vi "UPPub.vi"(8 "error in (no error)":errorcluster, 11 "GuiderSetup in":refnum<class "GuiderSetup.lvclass">) -> (0 "error out":errorcluster, 2 "STATUS cluster":T1, 3 "GuiderSetup out":refnum<class "GuiderSetup.lvclass">)   [LabVIEW 2018, in "GuiderSetup.lvclass"]
uses:
  GuiderSetup.lvclass
  C:/Users/observer/Desktop/Sparc4GUI/Versao ZeroMQ/SPARC4_GUI -20240706_20240708/S4GUI/S4GUI.lvclass
  S4GUI/S4GUI.lvclass/S4GUI.ctl
  Server/Server.lvclass/Server.ctl
  GuiderSetup.lvclass/GuiderSetup.ctl
  Instrument/Instrument.lvclass
  C:/Users/observer/Desktop/Sparc4GUI/Versao ZeroMQ/SPARC4_GUI -20240706_20240708/Server/Server.lvclass
  PublisherGS/PublisherGS.lvclass
  AG/AG.lvclass
  Server/Server.lvclass
  S4GUI/S4GUI.lvclass
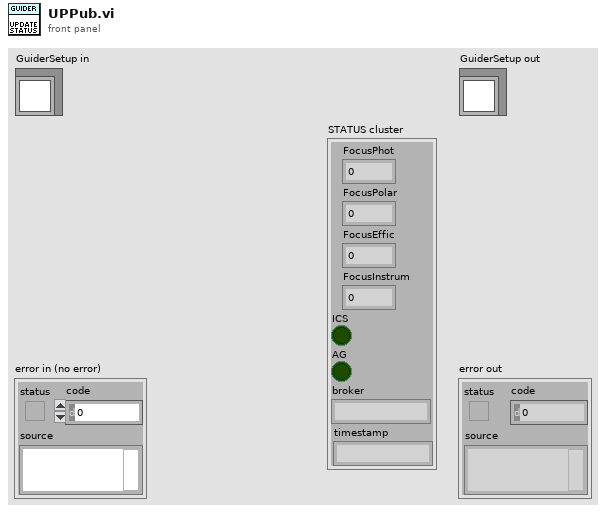
[diagram p1: front panel]
types:
  T1 = cluster{"FocusPhot":dbl, "FocusPolar":dbl, "FocusEffic":dbl, "FocusInstrum":dbl, "ICS":bool, "AG":bool, "broker":string, "timestamp":string}
  T2 = cluster{"Photometric":dbl, " Polarimetry":dbl, "Polarimetry \nEfficiency":dbl, "Instrumental polarization":dbl}
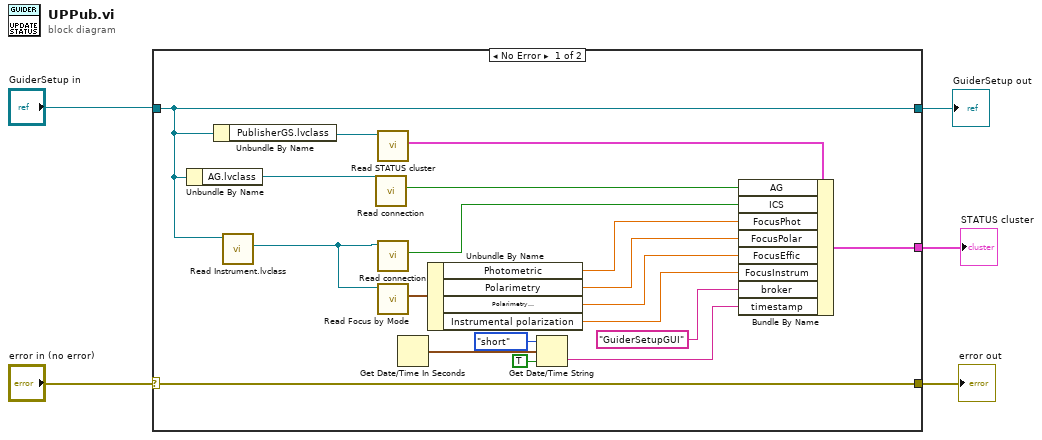
[diagram p0: block diagram]
diagram:
  n1 = case shown="No Error" "error in (no error)" {
    selector: "error in (no error)" -> [w10 w25]
    tunnel: [w19 w26] -> w2
    tunnel: "GuiderSetup in" -> [w19 w26]
    tunnel: [w24 _] -> w1
    tunnel: [w10 w25] -> w3
    frame No Error {
      n2 = Unbundle By Name(w19) -> ("AG.lvclass"=w21:refnum<class "AG.lvclass">)
      n3 = Unbundle By Name(w19) -> ("PublisherGS.lvclass"=w23:refnum<class "PublisherGS.lvclass">)
      n4 = call "Read Instrument.lvclass.vi"("S4ACS_GUI in"=w19) -> ("Instrument.lvclass"=w17:refnum<class "Instrument.lvclass">)  [unwired: 8 in, 2 out]
      n5 = call-dynamic "Read connection.vi"("Client in"=w21) -> ("connection"=w20:bool)  [unwired: 8 in, 2 out]
      n6 = call-dynamic "Read STATUS cluster.vi"("PublisherGS in"=w23) -> ("STATUS cluster"=w22:T1)  [unwired: 8 in, 2 out]
      n7 = call "Read connection.vi"("Server in"=w17) -> ("connection"=w18:bool)  [unwired: 8 in, 2 out]
      n8 = call-dynamic "Read Focus by Mode.vi"("Instrument in"=w17) -> ("Focus by Mode"=w16:T2)  [unwired: 8 in, 2 out]
      n9 = Get Date/Time In Seconds() -> (seconds since 1Jan1904=w6:timestamp)
      n10 = Unbundle By Name(w16) -> ("Photometric"=w14:dbl, "Polarimetry"=w13:dbl, "Polarimetry \nEfficiency"=w12:dbl, "Instrumental polarization"=w11:dbl)
      n11 = Get Date/Time String(date format (0)=enum16{"short", "long", "abbreviated"}."short", seconds (now)=w6, want seconds? (F)=TRUE) -> (time string=w9:string)  [unwired: 1 out]
      n12 = Bundle By Name(cluster=w22, "AG"=w20, "ICS"=w18, "FocusPhot"=w14, "FocusPolar"=w13, "FocusEffic"=w12, "FocusInstrum"=w11, "broker"="GuiderSetupGUI" ("BROKER"), "timestamp"=w9) -> (w24:T1)
    }
    frame Error {
    }
  }
  "error out" <- w3
  "GuiderSetup out" <- w2
  "STATUS cluster" <- w1
